vi "EF_GetFeaturesVectorAWT&Mean.vi"(8 "error in (no error)":errorcluster, 11 "Array Of Waveforms in":waveform(dbl)[](array[waveform])) -> (0 "error out":errorcluster, 3 "Features Array out":dbl[][](array[numeric]))   [LabVIEW 2016, in "Feature Extraction.lvlib"]
uses:
  <vilib>/addons/Wavelet Analysis/continuous wavelet transform.llb/WA Analytic Wavelet Transform (Waveform).vi
  Feature Extraction.lvlib
  <vilib>/addons/_Advanced Signal Processing/NI_AdvSigProcTFA.lvlib
  <vilib>/addons/_Advanced Signal Processing/NI_AdvSigProcWA.lvlib
  <vilib>/Analysis/NI_AALBase.lvlib
panel:
  # "This VI is a part of BCI Design library, http://www.ru-bci.org \nCopyright © 2020, Sotnikov Peter, All rights reserved. License: GNU GPLv3"
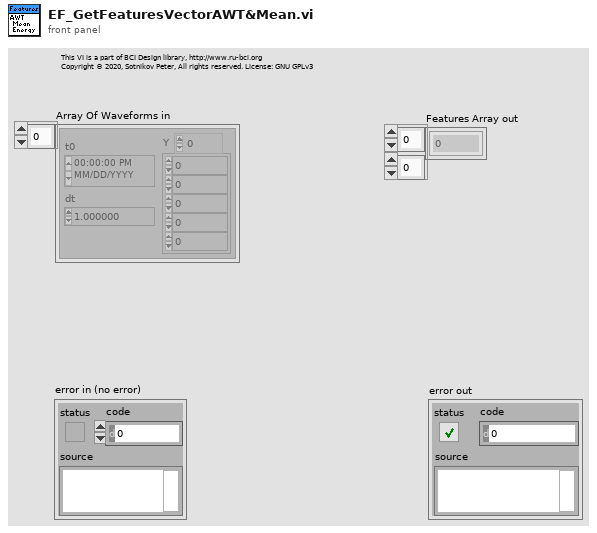
[diagram p1: front panel]
types:
  T1 = cluster{"frequency offset":dbl, "frequency multiplier":dbl}
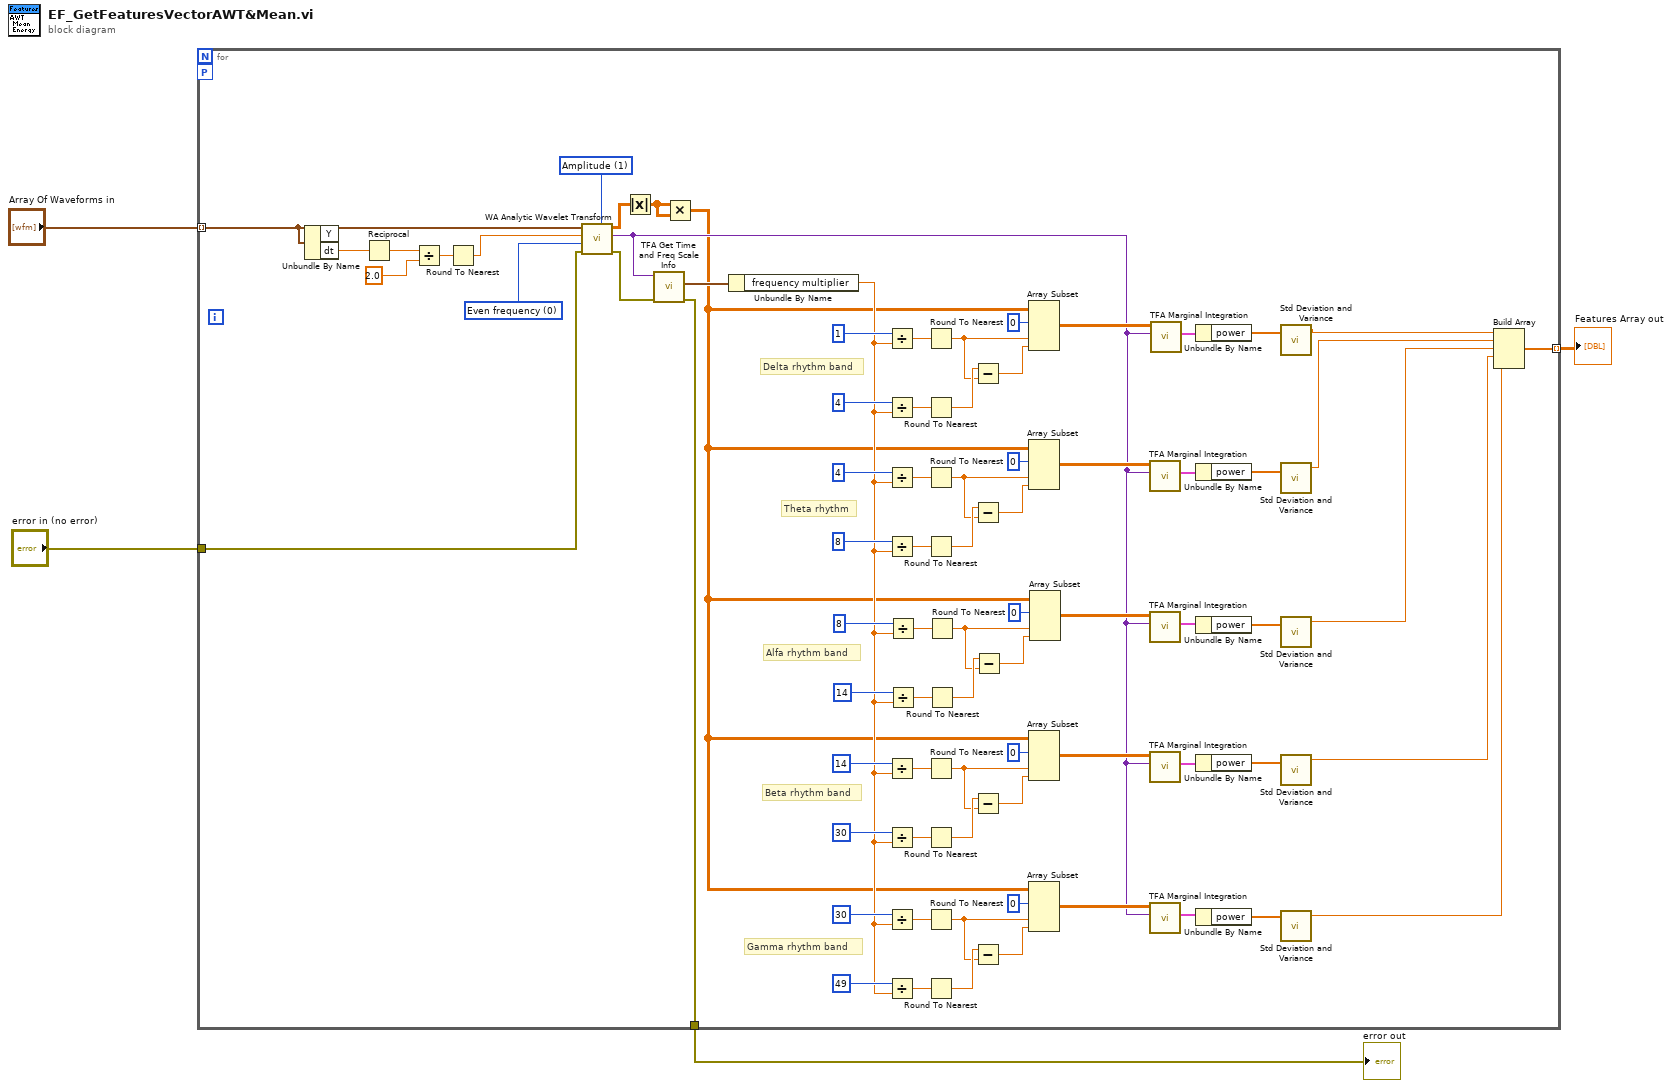
[diagram p0: block diagram]
diagram:
  n1 = for {
    tunnel: "error in (no error)" -> [w82]
    tunnel: [w38] -> w2 mode=indexing
    tunnel: [w37] -> w3
    tunnel: "Array Of Waveforms in" -> [w5] mode=indexing
    workers-P: _ -> [_]
    w29 = u16 0 items=["Even frequency", "Even scale"] ("scale sampling method")
    w30 = u16 1 items=["Energy", "Amplitude"] ("normalization")
    # "Gamma rhythm band"
    # "Beta rhythm band"
    # "Theta rhythm"
    # "Delta rhythm band"
    # "Alfa rhythm band"
    n2 = Unbundle By Name(w5) -> ("dt"=w26:dbl)  [unwired: 1 out]
    n3 = Reciprocal(x=w26) -> (1/x=w25:dbl)
    n4 = Divide(x=w25, y=2.0) -> (x/y=w23:dbl)
    n5 = Round To Nearest(number=w23) -> (nearest integer value=w22:dbl)
    n6 = call-poly <vilib>:"WA Analytic Wavelet Transform.vi"("normalization"=w30, "error in (no error)"=w82, "scale sampling method"=w29, "scales"=w22, "signal"=w5) -> ("error out"=w81:errorcluster, "scale info"=w31:variant, "AWT coef"=w28:cdb[][])  [unwired: 4 in]
    n7 = Absolute Value(x=w28) -> (abs(x)=w27:dbl[][])
    n8 = call <vilib>:"TFA Get Time and Freq Scale Info.vi"("error in (no error)"=w81, "scale info"=w31) -> ("error out"=w37:errorcluster, "frequency info"=w80:T1)  [unwired: 7 in, 1 out]
    n9 = Multiply(x=w27, y=w27) -> (x*y=w11:dbl[][])
    n10 = Unbundle By Name(w80) -> ("frequency multiplier"=w39:dbl)
    n11 = Divide(x=1, y=w39) -> (x/y=w79:dbl)
    n12 = Divide(x=4, y=w39) -> (x/y=w77:dbl)
    n13 = Divide(x=4, y=w39) -> (x/y=w71:dbl)
    n14 = Divide(x=8, y=w39) -> (x/y=w69:dbl)
    n15 = Divide(x=14, y=w39) -> (x/y=w55:dbl)
    n16 = Divide(x=30, y=w39) -> (x/y=w53:dbl)
    n17 = Divide(x=30, y=w39) -> (x/y=w47:dbl)
    n18 = Divide(x=49, y=w39) -> (x/y=w45:dbl)
    n19 = Divide(x=8, y=w39) -> (x/y=w63:dbl)
    n20 = Divide(x=14, y=w39) -> (x/y=w61:dbl)
    n21 = Round To Nearest(number=w79) -> (nearest integer value=w73:dbl)
    n22 = Round To Nearest(number=w77) -> (nearest integer value=w74:dbl)
    n23 = Round To Nearest(number=w71) -> (nearest integer value=w65:dbl)
    n24 = Round To Nearest(number=w69) -> (nearest integer value=w66:dbl)
    n25 = Round To Nearest(number=w55) -> (nearest integer value=w49:dbl)
    n26 = Round To Nearest(number=w53) -> (nearest integer value=w50:dbl)
    n27 = Round To Nearest(number=w47) -> (nearest integer value=w41:dbl)
    n28 = Round To Nearest(number=w45) -> (nearest integer value=w42:dbl)
    n29 = Round To Nearest(number=w63) -> (nearest integer value=w57:dbl)
    n30 = Round To Nearest(number=w61) -> (nearest integer value=w58:dbl)
    n31 = Subtract(x=w74, y=w73) -> (x-y=w72:dbl)
    n32 = Subtract(x=w66, y=w65) -> (x-y=w64:dbl)
    n33 = Subtract(x=w50, y=w49) -> (x-y=w48:dbl)
    n34 = Subtract(x=w42, y=w41) -> (x-y=w40:dbl)
    n35 = Subtract(x=w58, y=w57) -> (x-y=w56:dbl)
    n36 = Array Subset(array=w11, index (row)=0 ("index"), index (col)=w73, length (col)=w72) -> (w36:dbl[][])  [unwired: 1 in]
    n37 = Array Subset(array=w11, index (row)=0 ("index"), index (col)=w65, length (col)=w64) -> (w35:dbl[][])  [unwired: 1 in]
    n38 = Array Subset(array=w11, index (row)=0 ("index"), index (col)=w49, length (col)=w48) -> (w33:dbl[][])  [unwired: 1 in]
    n39 = Array Subset(array=w11, index (row)=0 ("index"), index (col)=w41, length (col)=w40) -> (w32:dbl[][])  [unwired: 1 in]
    n40 = Array Subset(array=w11, index (row)=0 ("index"), index (col)=w57, length (col)=w56) -> (w34:dbl[][])  [unwired: 1 in]
    n41 = call <vilib>:"TFA Marginal Integration.vi"("scale info"=w31, "spectrogram"=w35) -> ("time marginal integral"=w15:cluster{"t0":dbl, "dt":dbl, "power":dbl[]})  [unwired: 7 in, 2 out]
    n42 = call <vilib>:"TFA Marginal Integration.vi"("scale info"=w31, "spectrogram"=w34) -> ("time marginal integral"=w14:cluster{"t0":dbl, "dt":dbl, "power":dbl[]})  [unwired: 7 in, 2 out]
    n43 = call <vilib>:"TFA Marginal Integration.vi"("scale info"=w31, "spectrogram"=w33) -> ("time marginal integral"=w13:cluster{"t0":dbl, "dt":dbl, "power":dbl[]})  [unwired: 7 in, 2 out]
    n44 = call <vilib>:"TFA Marginal Integration.vi"("scale info"=w31, "spectrogram"=w32) -> ("time marginal integral"=w12:cluster{"t0":dbl, "dt":dbl, "power":dbl[]})  [unwired: 7 in, 2 out]
    n45 = call <vilib>:"TFA Marginal Integration.vi"("scale info"=w31, "spectrogram"=w36) -> ("time marginal integral"=w16:cluster{"t0":dbl, "dt":dbl, "power":dbl[]})  [unwired: 7 in, 2 out]
    n46 = Unbundle By Name(w16) -> ("power"=w20:dbl[])
    n47 = Unbundle By Name(w15) -> ("power"=w19:dbl[])
    n48 = Unbundle By Name(w14) -> ("power"=w18:dbl[])
    n49 = Unbundle By Name(w13) -> ("power"=w17:dbl[])
    n50 = Unbundle By Name(w12) -> ("power"=w21:dbl[])
    n51 = call <vilib>:"Std Deviation and Variance.vi"("X"=w20) -> ("mean"=w10:dbl)  [unwired: 1 in, 2 out]
    n52 = call <vilib>:"Std Deviation and Variance.vi"("X"=w19) -> ("mean"=w9:dbl)  [unwired: 1 in, 2 out]
    n53 = call <vilib>:"Std Deviation and Variance.vi"("X"=w18) -> ("mean"=w8:dbl)  [unwired: 1 in, 2 out]
    n54 = call <vilib>:"Std Deviation and Variance.vi"("X"=w17) -> ("mean"=w7:dbl)  [unwired: 1 in, 2 out]
    n55 = call <vilib>:"Std Deviation and Variance.vi"("X"=w21) -> ("mean"=w6:dbl)  [unwired: 1 in, 2 out]
    n56 = Build Array(w10, w9, w8, w7, w6) -> (w38:dbl[])
  }
  "Features Array out" <- w2
  "error out" <- w3
